vi "Add Section.vi"(4 "Property Values":variant[](array[variant]), 6 "Property names":string[](array[string]), 8 "error in (no error)":errorcluster, 9 "TypeGUID":string, 10 "SectionName":string, 11 "Section Reference in":u64 format="%.0x") -> (0 "error out":errorcluster, 1 "Newly Created?":bool, 2 "Section Reference":u64 format="%.0x", 3 "Section Reference out":u64 format="%.0x")   [LabVIEW 2013, in "Hierarchy Framework.lvlib" / "Section.lvclass"]
doc: "Adds a section with the name <B>Section Name</B> to the device specified by <B>Section Reference in</B>. If the <B>Section Name</B> you specify already exists for that device, this VI updates the values of any properties."
uses:
  Section.lvclass
  Generic/Generic.lvclass
  Item/Item.lvclass
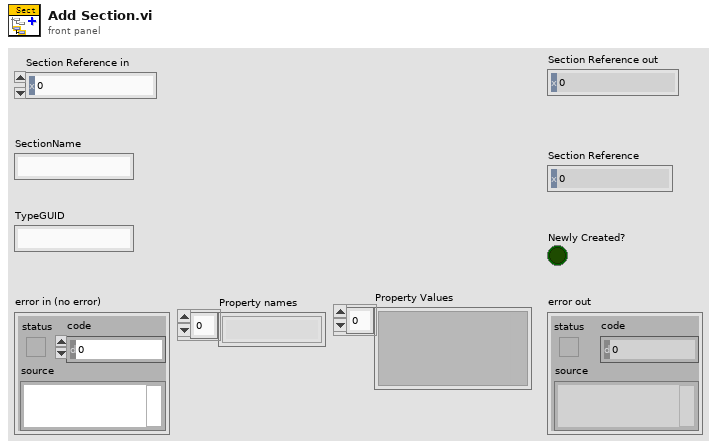
[diagram p1: front panel]
types:
  T1 = typedef "Hierarchy Framework.lvlib/Item.lvclass/Item Reference.ctl" = u64
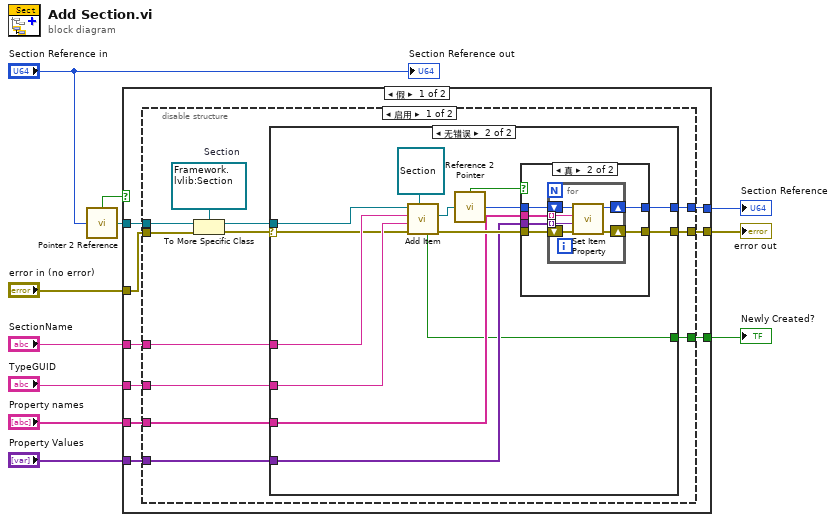
[diagram p0: block diagram]
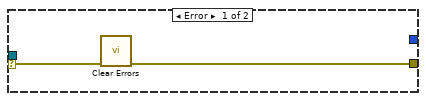
[diagram p2: hidden frame]
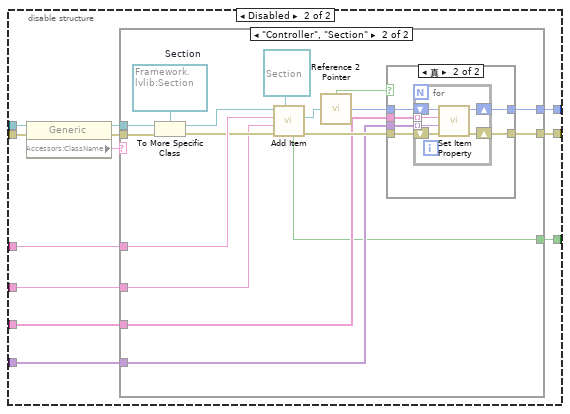
[diagram p4: hidden frame]
diagram:
  n1 = call "Pointer 2 Reference.vi"("Pointer"="Section Reference in") -> ("Not A Refnum?"=w5:bool, "Generic Reference"=w4:refnum<data-value>)
  n2 = case shown="假" w5 {
    tunnel: w4 -> [w16 _]
    tunnel: "SectionName" -> [w20 _]
    tunnel: "error in (no error)" -> [w15 w107]
    tunnel: [w17 _] -> w9
    tunnel: [w19 _] -> w8
    tunnel: [w18 w107] -> w7
    tunnel: "Property names" -> [w14 _]
    tunnel: "Property Values" -> [w13 _]
    tunnel: "TypeGUID" -> [w12 _]
    frame False {
      n3 = disable-structure shown="启用" {
        disable-tunnel: w20 -> [w32 w74]
        disable-tunnel: [w31 w73] -> w19
        disable-tunnel: [w30 w72] -> w18
        disable-tunnel: [w29 w71] -> w17
        disable-tunnel: w16 -> [w23 w70]
        disable-tunnel: w15 -> [w24 w66]
        disable-tunnel: w14 -> [w28 w65]
        disable-tunnel: w13 -> [w27 w64]
        disable-tunnel: w12 -> [w26 w63]
        frame Enabled {
          w25 = refnum<data-value> refnum  # Section
          n4 = To More Specific Class(target class=w25, reference=w23, error in=w24) -> (specific class reference=w21:refnum<data-value>, error out=w22:errorcluster)
          n5 = case shown="无错误" w22 {
            selector: w22 -> [w34 w36]
            tunnel: w32 -> [_ w48]
            tunnel: [_ w39] -> w31
            tunnel: [w33 w44] -> w30
            tunnel: [_ w45] -> w29
            tunnel: w28 -> [_ w43]
            tunnel: w27 -> [_ w42]
            tunnel: w26 -> [_ w37]
            tunnel: w21 -> [_ w35]
            frame Error {
              n6 = call <vilib>:"Clear Errors.vi"("error in (no error)"=w34) -> ("error out"=w33:errorcluster)  [unwired: 6 in]
            }
            frame No Error {
              n7 = call "Add Item.vi"("Type"=refnum<class "Section.lvclass"> refnum ("Framework.lvlib:Section"), "错误输入（无错误）"=w36, "TypeGUID"=w37, "Name"=w48, "Section in"=w35) -> ("错误输出"=w46:errorcluster, "Item"=w40:refnum<data-value>, "Newly Created?"=w39:bool)  [unwired: 3 in, 1 out]
              n8 = call "Reference 2 Pointer.vi"("Generic Reference"=w40) -> ("Valid?"=w41:bool, "Pointer"=w47:u64)
              n9 = case shown="真" w41 {
                tunnel: w47 -> [w50 w56]
                tunnel: w46 -> [w49 w55]
                tunnel: [w50 w54] -> w45
                tunnel: [w49 w53] -> w44
                tunnel: w43 -> [_ w52]
                tunnel: w42 -> [_ w51]
                frame False {
                }
                frame True {
                  n10 = for {
                    shift-right: [w60] -> w54
                    shift-left: w56 -> [w62]
                    shift-right: [w59] -> w53
                    shift-left: w55 -> [w61]
                    tunnel: w52 -> [w58] mode=indexing
                    tunnel: w51 -> [w57] mode=indexing
                    n11 = call "Set Item Property.vi"("error in (no error)"=w61, "Value"=w57, "Property Name"=w58, "Item Reference in"=w62) -> ("error out"=w59:errorcluster, "Item Reference out"=w60:T1)  [unwired: 5 in, 1 out]
                  }
                }
              }
            }
          }
        }
        frame Disabled {
          n12 = property class="Generic"(reference=w70, error in=w66) -> (reference out=w67:refnum<data-value>, error out=w68:errorcluster, "Accessors:ClassName"=w69:string)
          n13 = case shown="\"Controller\", \"Section\"" w69 {
            tunnel: w74 -> [_ w92]
            tunnel: [_ w78] -> w73
            tunnel: [w75 w83] -> w72
            tunnel: [_ w84] -> w71
            tunnel: w68 -> [w75 w88]
            tunnel: w67 -> [_ w87]
            tunnel: w65 -> [_ w82]
            tunnel: w64 -> [_ w81]
            tunnel: w63 -> [_ w76]
            frame "假", Default {
            }
            frame "Controller", "Section" {
              w90 = refnum<data-value> refnum  # Section
              n14 = To More Specific Class(target class=w90, reference=w87, error in=w88) -> (specific class reference=w89:refnum<data-value>, error out=w91:errorcluster)
              n15 = call "Add Item.vi"("Type"=refnum<class "Section.lvclass"> refnum ("Framework.lvlib:Section"), "错误输入（无错误）"=w91, "TypeGUID"=w76, "Name"=w92, "Section in"=w89) -> ("错误输出"=w85:errorcluster, "Item"=w79:refnum<data-value>, "Newly Created?"=w78:bool)  [unwired: 3 in, 1 out]
              n16 = call "Reference 2 Pointer.vi"("Generic Reference"=w79) -> ("Valid?"=w80:bool, "Pointer"=w86:u64)
              n17 = case shown="真" w80 {
                tunnel: w86 -> [w94 w100]
                tunnel: w85 -> [w93 w99]
                tunnel: [w94 w98] -> w84
                tunnel: [w93 w97] -> w83
                tunnel: w82 -> [_ w96]
                tunnel: w81 -> [_ w95]
                frame False {
                }
                frame True {
                  n18 = for {
                    shift-right: [w104] -> w98
                    shift-left: w100 -> [w106]
                    shift-right: [w103] -> w97
                    shift-left: w99 -> [w105]
                    tunnel: w96 -> [w102] mode=indexing
                    tunnel: w95 -> [w101] mode=indexing
                    n19 = call "Set Item Property.vi"("error in (no error)"=w105, "Value"=w101, "Property Name"=w102, "Item Reference in"=w106) -> ("error out"=w103:errorcluster, "Item Reference out"=w104:T1)  [unwired: 5 in, 1 out]
                  }
                }
              }
            }
          }
        }
      }
    }
    frame True {
    }
  }
  "Section Reference" <- w9
  "error out" <- w7
  "Newly Created?" <- w8
  "Section Reference out" <- "Section Reference in"
